vi "DSF.Memory.Pointer.U32.New.vi"(8 "error in (no error)":errorcluster, 11 "count":u64 format="%d elements") -> (0 "error out":errorcluster, 3 "pointer":refnum<class "DSF.Memory.Pointer.U32.lvclass">)   [LabVIEW 2016, in "DSF.Memory.lvlib" / "DSF.Memory.Pointer.U32.lvclass"]
uses:
  DSF.Memory.Pointer.U32.lvclass
  Submodules/Memory Manager/Source/Classes/Pointer/Memory.Pointer.lvclass/Memory.Pointer.ctl
  Submodules/Memory Manager/Source/Classes/Pointer/Accessors/Set Address.vi
  Submodules/Memory Manager/Source/Classes/Pointer/Accessors/Set Size.vi
  Submodules/Memory Manager/Source/Classes/Pointer.Internal/Memory.Pointer.Internal.lvclass
  C:/Git/SourceTree/data-sharing-framework/Source/Submodules/Memory Manager/Source/Classes/Pointer/Memory.Pointer.lvclass
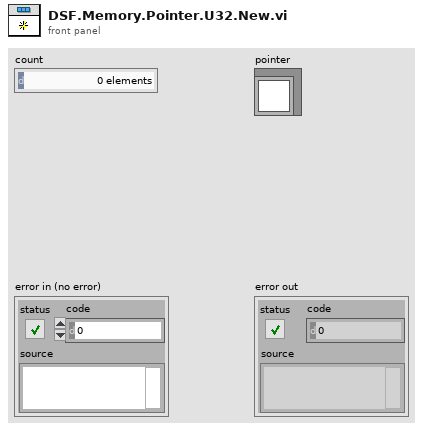
[diagram p1: front panel]
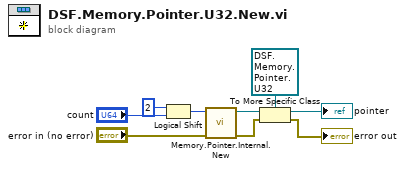
[diagram p0: block diagram]
diagram:
  n1 = Logical Shift(y=i16 2 ("power of 2"), x="count") -> (x << y=w1:u64)
  n2 = call "Memory.Pointer.Internal.New.vi"("error in (no error)"="error in (no error)", "size"=w1) -> ("error out"=w6:errorcluster, "pointer"=w8:refnum<class "Memory.Pointer.Internal.lvclass">)  [unwired: 8 in]
  n3 = To More Specific Class(target class=refnum<class "DSF.Memory.Pointer.U32.lvclass"> refnum ("DBL Pointer"), reference=w8, error in=w6) -> (specific class reference=→"pointer":refnum<class "DSF.Memory.Pointer.U32.lvclass">, error out=→"error out":errorcluster)
